vi "Header from Iteration.vi"(6 "frame_id":string="world", 10 "Rate (Hz)":dbl=1000.0 format="%#_13g", 11 "Iteration":i32) -> (3 "Header":T1)   [LabVIEW 2013]
uses:
  std_msgs/Header.ctl
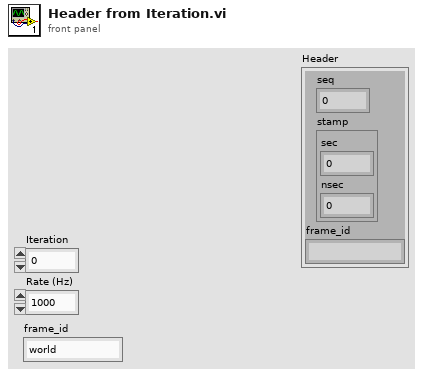
[diagram p1: front panel]
types:
  T1 = typedef "Header.ctl" = cluster{"seq":u32, "stamp":cluster{"sec":i32, "nsec":i32}, "frame_id":string}
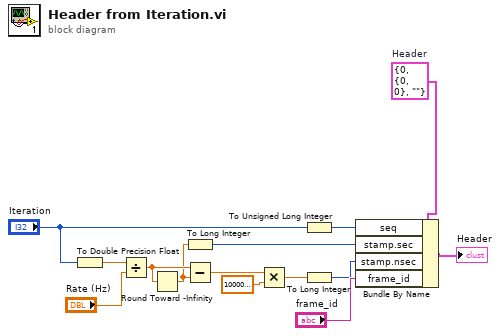
[diagram p0: block diagram]
diagram:
  w2 = T1 {"seq"=0, "stamp"={"sec"=0, "nsec"=0}, "frame_id"=""}  # Header
  n1 = To Double Precision Float(number="Iteration") -> (double precision float=w14:dbl)
  n2 = Divide(x=w14, y="Rate (Hz)") -> (x/y=w8:dbl)
  n3 = Round Toward -Infinity(1:w8) -> (0:w7:dbl)
  n4 = To Long Integer(number=w7) -> (32bit integer=w9:i32)
  n5 = Subtract(x=w8, y=w7) -> (x-y=w6:dbl)
  n6 = Multiply(x=w6, y=1000000000.0) -> (x*y=w4:dbl)
  n7 = To Unsigned Long Integer(number="Iteration") -> (unsigned 32bit integer=w11:u32)
  n8 = To Long Integer(number=w4) -> (32bit integer=w3:i32)
  n9 = Bundle By Name(cluster=w2, "seq"=w11, "stamp.sec"=w9, "stamp.nsec"=w3, "frame_id"="frame_id") -> (→"Header":T1)
